vi "fmt_GenerateExcelColumns_AA_AB.vi"(11 "NumColumns":i32) -> (3 "Column":string)   [LabVIEW 2017, in "NI_ExcelFile.lvlib"]
uses:
  <vilib>/express/express shared/NI_ExcelFile/NI_ExcelFile.lvlib
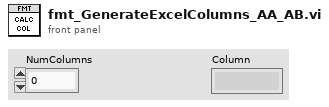
[diagram p1: front panel]
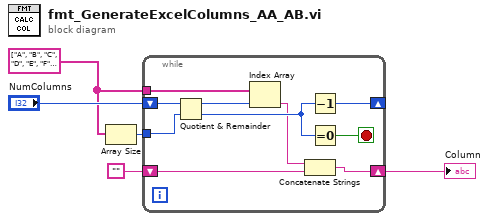
[diagram p0: block diagram]
diagram:
  w4 = string[] ["A", "B", "C", "D", "E", "F", "G", "H", "I", "J", "K", "L", "M", "N", "O", "P", "Q", "R", "S", "T", "U", "V", "W", "X", "Y", "Z"]
  n1 = Array Size(array=w4) -> (size(s)=w3:i32)
  n2 = while {
    shift-right: [w13] -> _
    shift-left: "NumColumns" -> [w15]
    tunnel: w4 -> [w9]
    tunnel: w3 -> [w14]
    shift-right: [w8] -> w1
    shift-left: "" -> [w7]
    stop <- w12 stop-if-true
    n3 = Quotient & Remainder(x=w15, y=w14) -> (x-y*floor(x/y)=w10:i32, floor(x/y)=w11:i32)
    n4 = Index Array(array=w9, index=w10) -> (element=w6:string)
    n5 = Concatenate Strings(w6, w7) -> (w8:string)
    n6 = Decrement(x=w11) -> (x-1=w13:i32)
    n7 = Equal To 0?(x=w11) -> (x = 0?=w12:bool)
  }
  "Column" <- w1
